vi "Typecast Queue to Refnum.vi"(11 "queue in":refnum<queue>) -> (3 "refnum out":T1)   [LabVIEW 2014, in "Raspberry Pi Compatible Compiler for LabVIEW.lvlib"]
uses:
  Raspberry Pi Compatible Compiler for LabVIEW.lvlib
  <vilib>/Utility/config.llb/Config Data RefNum.ctl
  TypeDefs/Config Data.ctl
  TypeDefs/Section.ctl
  TypeDefs/Config Data RefNum.ctl
  <vilib>/Utility/config.llb/NI_LVConfig.lvlib
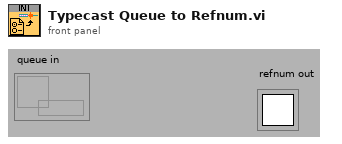
[diagram p1: front panel]
types:
  T1 = typedef "NI_LVConfig.lvlib/Config Data RefNum.ctl" = refnum<k1>
  T2 = typedef "Raspberry Pi Compatible Compiler for LabVIEW.lvlib/Config Data RefNum.ctl" = refnum<k1>
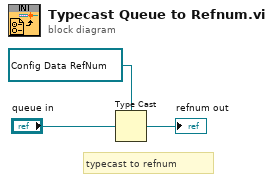
[diagram p0: block diagram]
diagram:
  w2 = T2 refnum items=["config data"] ("refnum out")
  # "typecast to refnum"
  n1 = Type Cast(type=w2, x="queue in") -> (*(type *) &x=→"refnum out":T2)
